vi "SailAndRudderArbiter.vi"(0 "WindToSailLookup":dbl, 1 "TackingSailSuggestion":dbl, 5 "BalanceRudderSailSugggestion":dbl, 7 "TurtleModeSailSuggestion":dbl, 9 "LuffToSailSuggestion":dbl, 11 "TurningSailSuggestion":dbl, 12 "JibeSailSuggestion":dbl) -> (4 "MainSailSetpoint":dbl, 6 "JibSetpoint":dbl, 10 "Rudder Setpoint":dbl)   [LabVIEW 2012]
panel:
  in  "TimeOnThisState":i32
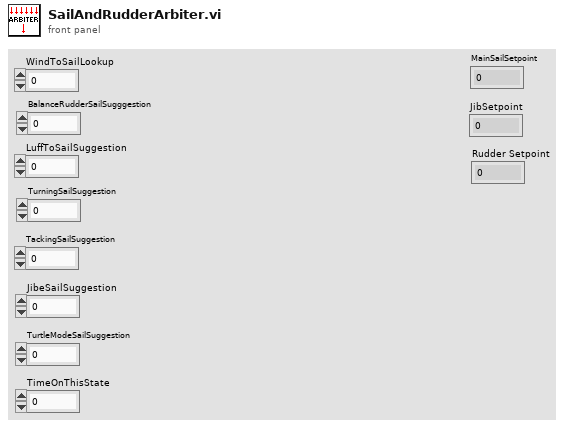
[diagram p1: front panel]
types:
  T1 = typedef "Sailing State of Boat.ctl" = enum16{"Straight", "Turning", "Approach Maneuver", "Cross Wind (Tack)", "Cross Wind (Gybe)", "Turtle Mode", ""}
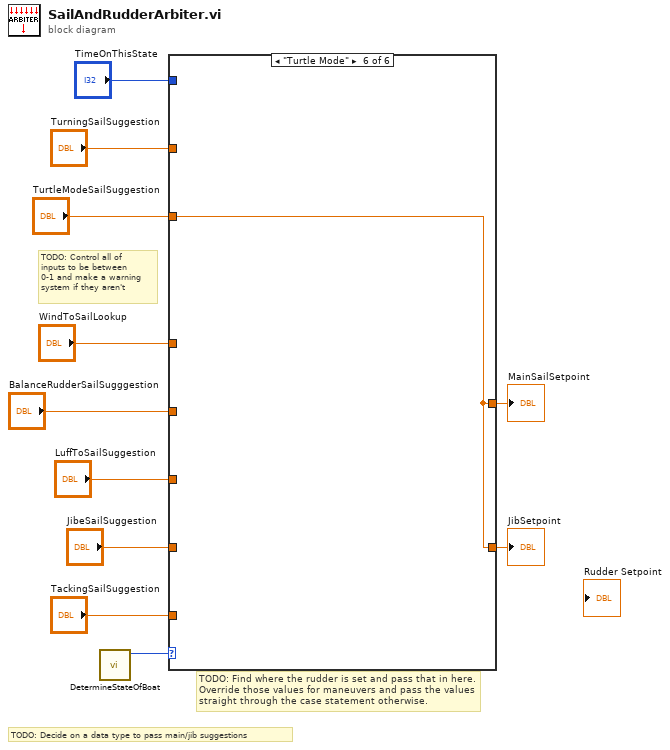
[diagram p0: block diagram]
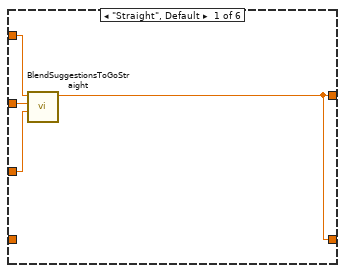
[diagram p2: hidden frame]
diagram:
  # "TODO: Find where the rudder is set and pass that in here.\nOverride those values for maneuvers and pass the values\nstraight through the case statement otherwise."
  # "TODO: Decide on a data type to pass main/jib suggestions"
  # "TODO: Control all of\ninputs to be between\n0-1 and make a warning\nsystem if they aren't"
  n1 = call "DetermineStateOfBoat.vi"() -> ("StateOfBoat"=w1:T1)  [unwired: 9 in, 1 out]
  n2 = case shown="\"Turtle Mode\"" w1 {
    tunnel: [w12 w16 w17 w18 w19 w20] -> w11
    tunnel: [w12 w16 w17 w18 w19 w20] -> w10
    tunnel: "JibeSailSuggestion" -> [_ _ _ _ w19 _]
    tunnel: "TackingSailSuggestion" -> [_ _ _ w18 _ _]
    tunnel: "WindToSailLookup" -> [w15 _ w17 _ _ _]
    tunnel: "TurningSailSuggestion" -> [_ w16 _ _ _ _]
    tunnel: "TimeOnThisState" -> [_ _ _ _ _ _]
    tunnel: "TurtleModeSailSuggestion" -> [_ _ _ _ _ w20]
    tunnel: "BalanceRudderSailSugggestion" -> [w14 _ _ _ _ _]
    tunnel: "LuffToSailSuggestion" -> [w13 _ _ _ _ _]
    frame "Straight", Default {
      n3 = call "BlendSuggestionsToGoStraight.vi"("LuffToSailSuggestion"=w13, "BalanceRudderSailSuggestion"=w14, "WindToSailLookup"=w15) -> ("BlendedSailSuggestion"=w12:dbl)  [unwired: 8 in]
    }
    frame "Turning" {
    }
    frame "Approach Maneuver" {
    }
    frame "Cross Wind (Tack)" {
      # "Use the tack suggestions here!"
    }
    frame "Cross Wind (Gybe)" {
      # "Use the jibe suggestions here!"
    }
    frame "Turtle Mode" {
    }
  }
  "MainSailSetpoint" <- w11
  "JibSetpoint" <- w10
